vi "Final Max & Min Array without using array.vi"() -> ()   [LabVIEW 2020]
panel:
  out "Numeric 2":i32
  out "Numeric":i32
  in  "stop":bool
  out "MIN":dbl
  out "MAX":dbl
  in  "Array":dbl[](array[numeric])
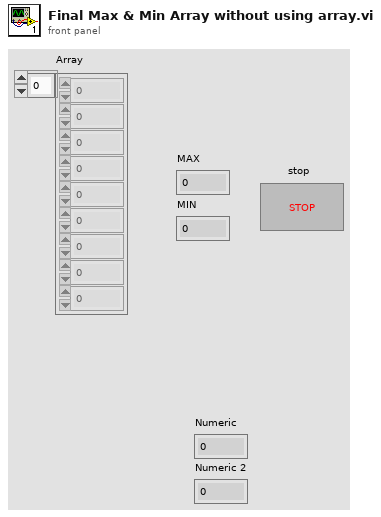
[diagram p1: front panel]
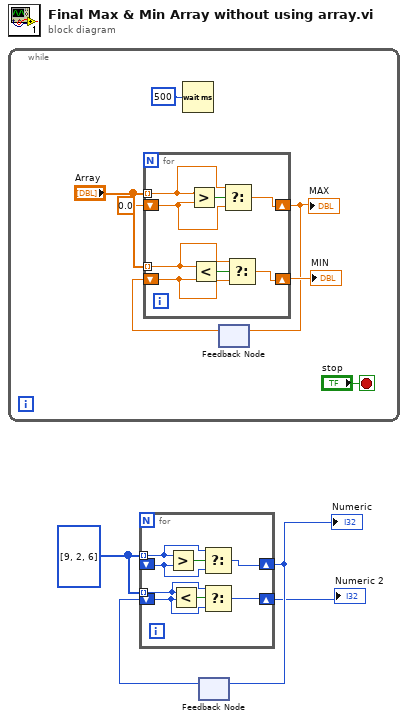
[diagram p0: block diagram]
diagram:
  w4 = i32[] [9, 2, 6]
  n1 = while {
    stop <- "stop" stop-if-true
    n2 = Wait (ms)(milliseconds to wait=u32 500) -> ()  [unwired: 1 out]
    n3 = feedback #1() -> (w8:dbl)  [unwired: 1 in]
    n4 = for {
      tunnel: "Array" -> [w16] mode=indexing
      shift-right: [w17] -> w9
      shift-left: 0.0 ("Numeric") -> [w15]
      tunnel: "Array" -> [w13] mode=indexing
      shift-right: [w14] -> w10
      shift-left: w8 -> [w12]
      n5 = Greater?(x=w16, y=w15) -> (0:w19:bool)
      n6 = Less?(x=w13, y=w12) -> (x < y?=w18:bool)
      n7 = Select(t=w16, s=w19, f=w15) -> (s? t:f=w17:dbl)
      n8 = Select(t=w13, s=w18, f=w12) -> (s? t:f=w14:dbl)
    }
    "MAX" <- w9
    "MIN" <- w10
    n9 = feedback-in #1(w9) -> ()
  }
  n10 = feedback #2() -> (w2:i32)  [unwired: 1 in]
  n11 = for {
    tunnel: w4 -> [w21] mode=indexing
    shift-right: [w25] -> w3
    shift-left: _ -> [w20]
    tunnel: w4 -> [w23] mode=indexing
    shift-right: [w24] -> w1
    shift-left: w2 -> [w22]
    n12 = Greater?(x=w21, y=w20) -> (0:w27:bool)
    n13 = Less?(x=w23, y=w22) -> (x < y?=w26:bool)
    n14 = Select(t=w21, s=w27, f=w20) -> (s? t:f=w25:i32)
    n15 = Select(t=w23, s=w26, f=w22) -> (s? t:f=w24:i32)
  }
  "Numeric" <- w3
  "Numeric 2" <- w1
  n16 = feedback-in #2(w3) -> ()
